vi "Write Name.vi"(8 "error in (no error)":errorcluster, 10 "Name":string, 11 "VI Info Data in":refnum<class "VI Info Data.lvclass">) -> (0 "error out":errorcluster, 3 "VI Info Data out":refnum<class "VI Info Data.lvclass">)   [LabVIEW 2020, in "VI Info Data.lvclass"]
uses:
  VI Info Data.lvclass
  VI Info Data.lvclass/VI Info Data.ctl
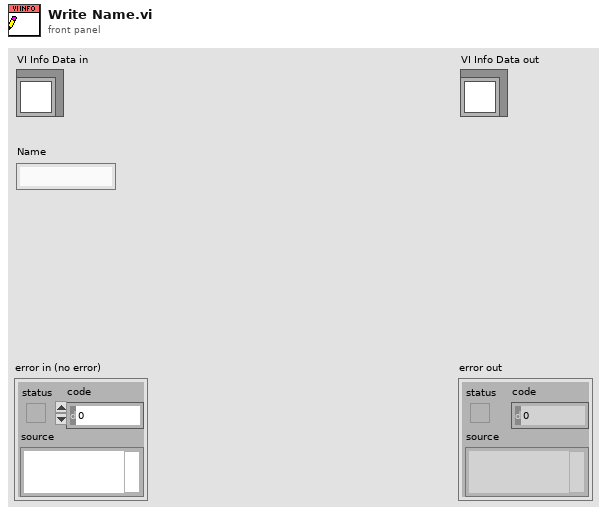
[diagram p1: front panel]
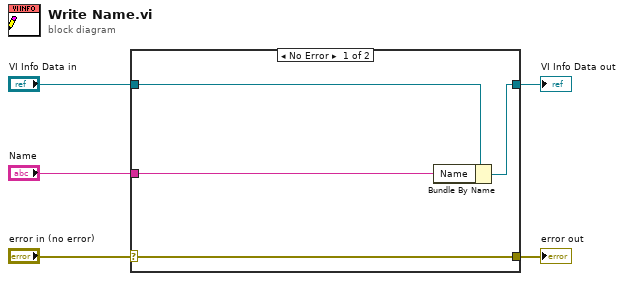
[diagram p0: block diagram]
diagram:
  n1 = case shown="No Error" "error in (no error)" {
    selector: "error in (no error)" -> [w9 w10]
    tunnel: [w9 w10] -> w4
    tunnel: [w7 w11] -> w2
    tunnel: "VI Info Data in" -> [w8 w11]
    tunnel: "Name" -> [w6 _]
    frame No Error {
      n2 = Bundle By Name(cluster=w8, "Name"=w6) -> (w7:refnum<class "VI Info Data.lvclass">)
    }
    frame Error {
    }
  }
  "error out" <- w4
  "VI Info Data out" <- w2
